vi "Write Token.vi"(8 "error in (no error)":errorcluster, 10 "Token":string, 11 "ByteRESTBase in":refnum<class "ByteRESTBase.lvclass">) -> (0 "error out":errorcluster, 3 "ByteRESTBase out":refnum<class "ByteRESTBase.lvclass">)   [LabVIEW 2019, in "ByteREST.lvlib" / "ByteRESTBase.lvclass"]
uses:
  ByteRESTBase.lvclass
  ByteRESTBase.lvclass/ByteRESTBase.ctl
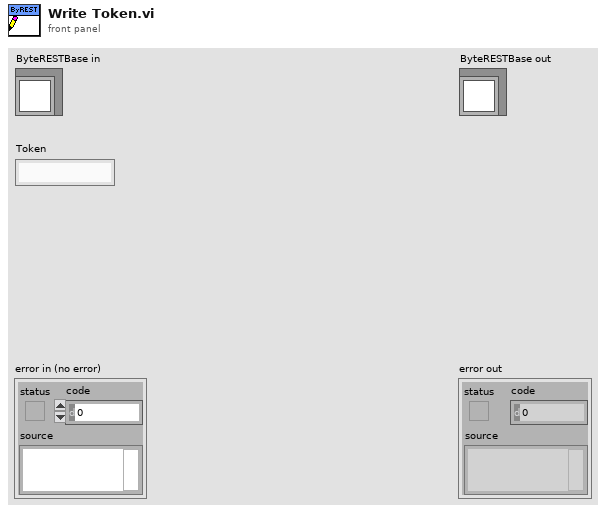
[diagram p1: front panel]
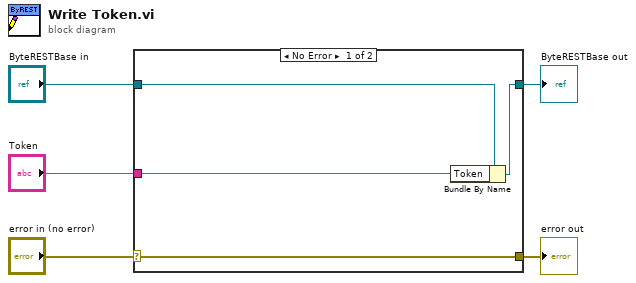
[diagram p0: block diagram]
diagram:
  n1 = case shown="No Error" "error in (no error)" {
    selector: "error in (no error)" -> [w9 w10]
    tunnel: [w9 w10] -> w4
    tunnel: [w7 w11] -> w2
    tunnel: "ByteRESTBase in" -> [w8 w11]
    tunnel: "Token" -> [w6 _]
    frame No Error {
      n2 = Bundle By Name(cluster=w8, "Token"=w6) -> (w7:refnum<class "ByteRESTBase.lvclass">)
    }
    frame Error {
    }
  }
  "error out" <- w4
  "ByteRESTBase out" <- w2
